vi "Convert_dBm_to_Watts.vi"(11 "P(dBm)":dbl[](array[numeric])) -> (3 "P(n_watts)":dbl[](array[numeric]))   [LabVIEW 2018]
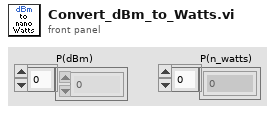
[diagram p1: front panel]
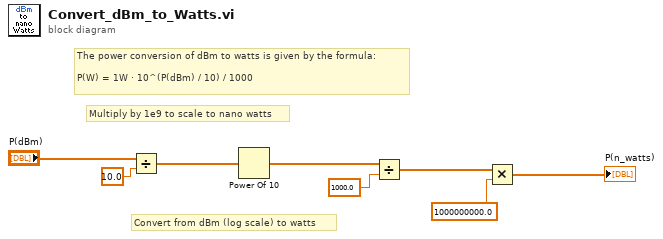
[diagram p0: block diagram]
diagram:
  # "Multiply by 1e9 to scale to nano watts"
  # "Convert from dBm (log scale) to watts"
  # "The power conversion of dBm to watts is given by the formula:\n\nP(W) = 1W · 10^(P(dBm) / 10) / 1000"
  n1 = Divide(x="P(dBm)", y=10.0) -> (x/y=w5:dbl[])
  n2 = Power Of 10(x=w5) -> (10^x=w6:dbl[])
  n3 = Divide(x=w6, y=1000.0) -> (x/y=w8:dbl[])
  n4 = Multiply(x=w8, y=1000000000.0) -> (x*y=→"P(n_watts)":dbl[])
